vi "save_data.vi"(1 "error in (no error)":errorcluster caption="错误输入（无错误）", 2 "Data":string[][](array[string]), 3 "数据文件路径":path caption="路径") -> (0 "error out":errorcluster caption="错误输出")   [LabVIEW 2018]
uses:
  <vilib>/Utility/NIReport.llb/Report Type.ctl
  <vilib>/Utility/NIReport.llb/Append Text Table to Report (wrap).vi
  <vilib>/Utility/NIReport.llb/NI_report.lvclass
  <vilib>/Utility/NIReport.llb/NI_ReportGenerationCore.lvlib
  <vilib>/Utility/NIReport.llb/Excel/NI_Excel.lvclass
types:
  T1 = typedef "NI_ReportGenerationCore.lvlib/Report Type.ctl" = enum16{"HTML", "Word", "Excel"}
  T2 = enum16{"maximized", "minimized", "normal", "no change"}
  T3 = cluster{"position (excel)":cluster{"row":i32, "column":i32}, "name (excel)":string, "bookmark (word)":string}
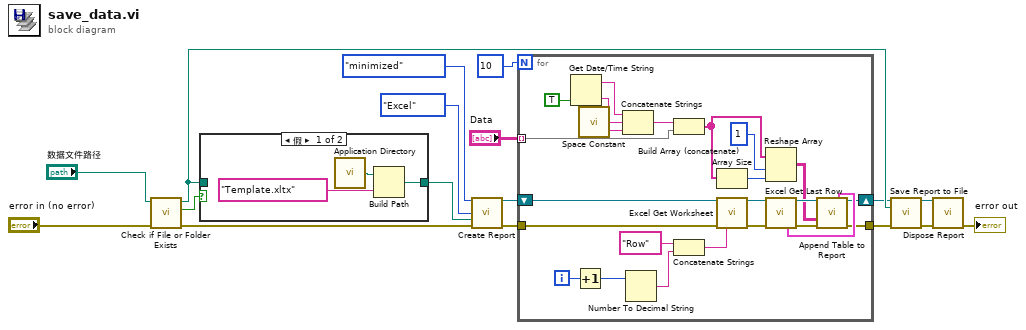
[diagram p0: block diagram]
diagram:
  n1 = call <vilib>:"Check if File or Folder Exists.vi"("error in (no error)"="error in (no error)", "path"="数据文件路径") -> ("error out"=w13:errorcluster, "file or folder exists?"=w17:bool, "dup path"=w8:path)  [unwired: 7 in]
  n2 = case shown="假" w17 {
    tunnel: w8 -> [_ w21]
    tunnel: [w19 w21] -> w14
    frame False {
      n3 = call <vilib>:"Application Directory.vi"() -> ("Application Directory"=w18:path)
      n4 = Build Path(base path=w18, name or relative path="Template.xltx" ("名称或相对路径")) -> (appended path=w19:path)
    }
    frame True {
    }
  }
  n5 = call <vilib>:"Create Report.vi"("window state (normal)"=T2."minimized", "report type"=Report_Type."Excel", "template (empty)"=w14, "error in (no error)"=w13) -> ("report out"=w10:refnum<class "NI_report.lvclass">, "error out"=w9:errorcluster)  [unwired: 10 in]
  n6 = for {
    N: 10 -> [_]
    tunnel: w9 -> [w39]
    tunnel: [w37] -> w4
    tunnel: "Data" -> [w30] mode=indexing
    shift-right: [w38] -> w5
    shift-left: w10 -> [w40]
    i -> [w28]
    n7 = Get Date/Time String(want seconds? (F)=TRUE ("需要秒？(F)")) -> (date string=w32:string, time string=w34:string)  [unwired: 2 in]
    n8 = Increment(x=w28) -> (x+1=w27:i32)
    n9 = call <vilib>:"Space Constant.vi"() -> ("String"=w33:string)
    n10 = Concatenate Strings(w32, w33, w34) -> (w35:string)
    n11 = Number To Decimal String(number=w27) -> (decimal integer string=w26:string)  [unwired: 1 in]
    n12 = Build Array (concatenate)(w35, w30) -> (w36:string[])
    n13 = Concatenate Strings("Row", w26) -> (w25:string)
    n14 = Array Size(array=w36) -> (size(s)=w24:i32)
    n15 = call <vilib>:"Excel Get Worksheet.vi"("report in"=w40, "error in (no error)"=w39, "name (\"\")"=w25) -> ("report out"=w45:refnum<class "NI_report.lvclass">, "error out"=w44:errorcluster)  [unwired: 11 in]
    n16 = Reshape Array(w36, 1 ("维数大小"), w24) -> (w22:string[][])
    n17 = call <vilib>:"Excel Get Last Row.vi"("report in"=w45, "error in (no error)"=w44) -> ("report out"=w43:refnum<class "NI_report.lvclass">, "MS Office parameters out"=w42:T3, "error out"=w41:errorcluster)  [unwired: 11 in]
    n18 = call-poly <vilib>:"Append Table to Report.vi"("report in"=w43, "MS Office parameters"=w42, "text data"=w22, "error in (no error)"=w41) -> ("report out"=w38:refnum<class "NI_report.lvclass">, "error out"=w37:errorcluster)  [unwired: 8 in, 2 out]
  }
  n19 = call-dynamic "Save Report to File.vi"("report in"=w5, "report file path"=w8, "error in (no error)"=w4) -> ("report out"=w6:refnum<class "NI_report.lvclass">, "error out"=w7:errorcluster)  [unwired: 11 in]
  n20 = call-dynamic "Dispose Report.vi"("report in"=w6, "error in (no error)"=w7) -> ("error out"=→"error out":errorcluster)  [unwired: 13 in]
